vi "Find Next True.vi"(2 "day of week":i32, 3 "Accessors:DoW":bool[](array[boolean])) -> (1 "index of element":i32)   [LabVIEW 2020, in "Daily.lvclass"]
uses:
  Daily/Daily.lvclass
  Daily/Daily.lvclass/Daily.ctl
  6432176b-51b5-44e0-b47b-c9ebaa285b2a.vi
  17329017-3dc8-47c8-aa80-4c5ed815302a.vi
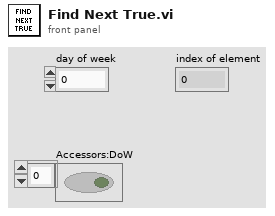
[diagram p1: front panel]
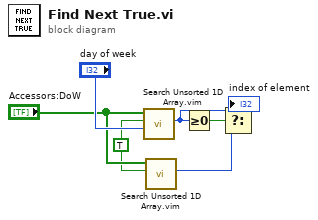
[diagram p0: block diagram]
diagram:
  w3 = TRUE
  n1 = call "Search Unsorted 1D Array.vim"("start index (0)"="day of week", "element"=w3, "unsorted 1D array"="Accessors:DoW") -> ("index of element"=w2:i32)  [unwired: 8 in]
  n2 = call "Search Unsorted 1D Array.vim"("element"=w3, "unsorted 1D array"="Accessors:DoW") -> ("index of element"=w5:i32)  [unwired: 9 in]
  n3 = Greater Or Equal To 0?(x=w2) -> (x >= 0?=w1:bool)
  n4 = Select(t=w2, s=w1, f=w5) -> (s? t:f=→"index of element":i32)
